vi "Q_Delete.vi"(8 "error in":errorcluster caption="错误输入（无错误）", 10 "CloseVI?(T)":bool=TRUE, 11 "ChildNode*":refnum<data-value>) -> (0 "error out":errorcluster caption="错误输出")   [LabVIEW 2013, in "PanelDataNode.lvclass"]
uses:
  PanelDataNode.lvclass
  PanelDataNode.lvclass/PanelDataNode.ctl
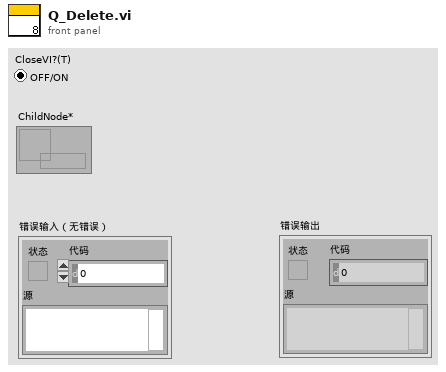
[diagram p1: front panel]
types:
  T1 = cluster{"ChildNode*":refnum<data-value>, "CloseVI?(T)":bool}
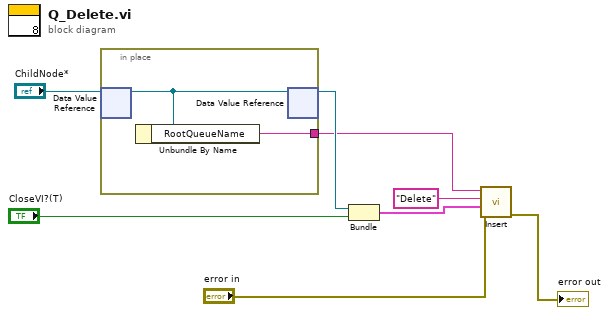
[diagram p0: block diagram]
diagram:
  n1 = in-place {
    in-place-border: [w9] -> w4
    n2 = in-place-dvr #1("ChildNode*") -> (w10:refnum<class "PanelDataNode.lvclass">)  [unwired: 1 out]
    n3 = Unbundle By Name(w10) -> ("RootQueueName"=w9:string)
    n4 = in-place-dvr #1(w10) -> (w5:refnum<data-value>)  [unwired: 1 out]
  }
  n5 = Bundle("ChildNode*"=w5, "CloseVI?(T)"="CloseVI?(T)") -> (w8:T1)  [unwired: 1 in]
  n6 = call "Insert.vi"("error in"="error in", "Data"=w8, "Event"="Delete", "QueueName"=w4) -> ("error out"=→"error out":errorcluster)  [unwired: 6 in, 1 out]
